vi "gu_open_file_dialog.vi"(7 "Prompt":T1, 8 "error in":errorcluster) -> (0 "error out":errorcluster, 2 "Cancelled":bool, 3 "Encoded Path":T1)   [LabVIEW 2020, in "G-Unicode.lvlib"]
uses:
  G-Unicode.lvlib
  Types/Encoded UTF-8 String.ctl
  Memory/Copy String.vi/4d47babd-4a2d-4eb7-b91b-7e707d692665.vi
  gu_free.vi
  <vilib>/Utility/file.llb/Application Directory.vi
  lib/g_unicode_32.dll
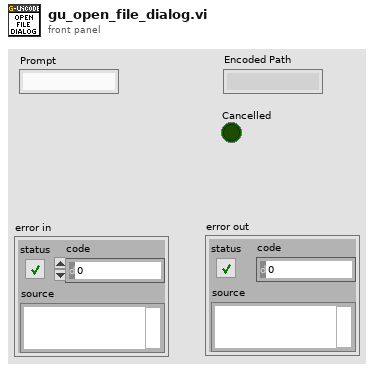
[diagram p1: front panel]
types:
  T1 = typedef "G-Unicode.lvlib/Encoded UTF-8 String.ctl" = string
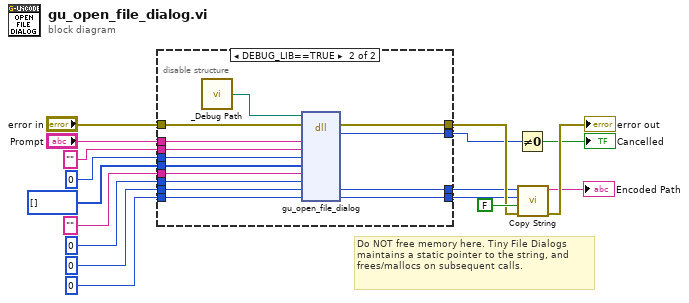
[diagram p0: block diagram]
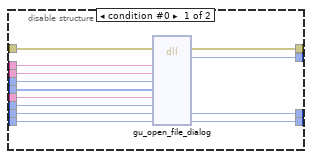
[diagram p2: hidden frame]
diagram:
  # "Do NOT free memory here. Tiny File Dialogs maintains a static pointer to the string, and frees/mallocs on subsequent calls."
  n1 = disable-structure shown="DEBUG_LIB==TRUE" {
    disable-tunnel: "error in" -> [w30 w44]
    disable-tunnel: [w29 w43] -> w12
    disable-tunnel: "Prompt" -> [w28 w42]
    disable-tunnel: "" ("default_path") -> [w27 w41]
    disable-tunnel: 0 ("num_filter_patterns") -> [w26 w40]
    disable-tunnel: i64[] [] ("filter_patterns") -> [w25 w39]
    disable-tunnel: "" ("filter_description") -> [w24 w38]
    disable-tunnel: 0 ("allow_multi_select") -> [w23 w37]
    disable-tunnel: i64 0 ("path_pointer") -> [w22 w36]
    disable-tunnel: 0 ("path_length") -> [w21 w35]
    disable-tunnel: [w20 w34] -> w11
    disable-tunnel: [w19 w33] -> w10
    disable-tunnel: [w18 w32] -> w9
    frame condition #0 {
      n2 = dll-call lib="C:/github/dataflowg/g-unicode/src/LabVIEW/G-Unicode/lib/g_unicode_*.*" fn="gu_open_file_dialog"(error in=w30, "title"=w28, "default_path"=w27, "num_filter_patterns"=w26, "filter_patterns"=w25, "filter_description"=w24, "allow_multi_select"=w23, "path_pointer"=w22, "path_length"=w21) -> (error out=w29:errorcluster, "return type"=w18:i32, "path_pointer"=w20:i64, "path_length"=w19:i32)  [unwired: 8 in, 1 out]
    }
    frame condition #1 (active) {
      n3 = call "_Debug Path.vi"() -> ("Debug Path"=w31:path)
      n4 = dll-call lib="?" fn="gu_open_file_dialog"(path in=w31, error in=w44, "title"=w42, "default_path"=w41, "num_filter_patterns"=w40, "filter_patterns"=w39, "filter_description"=w38, "allow_multi_select"=w37, "path_pointer"=w36, "path_length"=w35) -> (error out=w43:errorcluster, "return type"=w32:i32, "path_pointer"=w34:i64, "path_length"=w33:i32)  [unwired: 7 in, 1 out]
    }
  }
  n5 = Not Equal To 0?(x=w9) -> (x != 0?=→"Cancelled":bool)
  n6 = call "Copy String.vi"("error in"=w12, "free (F)"=FALSE, "size"=w10, "pointer"=w11) -> ("error out"=→"error out":errorcluster, "string"=→"Encoded Path":string)  [unwired: 6 in]
